vi "Msg.vi"(7 "Actor in":refnum<class "Actor.lvclass">, 11 "Actor Create Msg Strategy in":refnum<class "Actor Create Msg Strategy.lvclass">) -> (5 "Actor out":refnum<class "Actor.lvclass">)   [LabVIEW 2021, in "Actor Create.lvlib" / "Actor Create Msg Strategy.lvclass"]
uses:
  Actor Create Msg Strategy.lvclass
  jettl/Actor/Actor.lvclass
  Actor Create/Actor Create.lvclass
  b9b3c3c6-ce11-415e-ad89-e7059c446d1f.vi
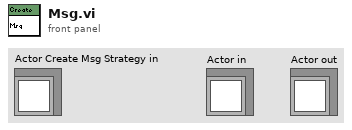
[diagram p1: front panel]
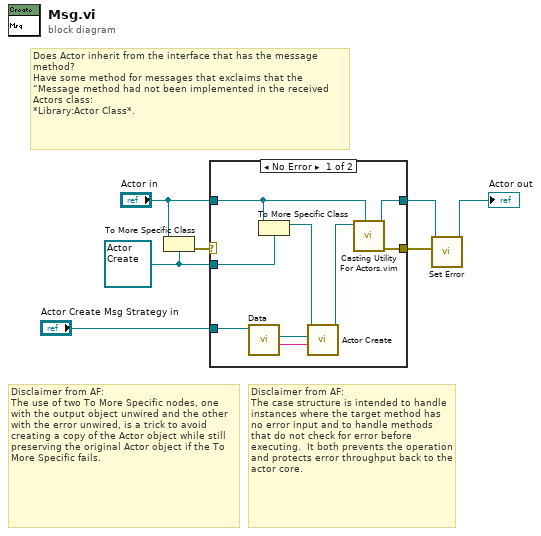
[diagram p0: block diagram]
diagram:
  w6 = refnum<class "Actor Create.lvclass"> refnum ("Create.lvlib:Create.lvclass")
  # "Disclaimer from AF:\nThe use of two To More Specific nodes, one with the output object unwired and the other with the error unwired, is a trick to avoid creating a copy of the Actor object while still preserving the original Actor object if the To More Specific fails."
  # "Disclaimer from AF:\nThe case structure is intended to handle instances where the target method has no error input and to handle methods that do not check for error before executing.  It both prevents the operation and protects error throughput back to the actor core."
  # "Does Actor inherit from the interface that has the message method?\nHave some method for messages that exclaims that the “Message method had not been implemented in the received Actors class:\n*Library:Actor Class*."
  n1 = To More Specific Class(target class=w6, reference="Actor in") -> (error out=w7:errorcluster)  [unwired: 1 in, 1 out]
  n2 = case shown="No Error" w7 {
    selector: w7 -> [_ w17]
    tunnel: [w13 w18] -> w2
    tunnel: "Actor in" -> [w12 w18]
    tunnel: w6 -> [w15 _]
    tunnel: "Actor Create Msg Strategy in" -> [w11 _]
    tunnel: [w8 w17] -> w3
    frame No Error {
      n3 = call "Data.vi"("Actor Create Msg Strategy in"=w11) -> ("Nested Alias"=w9:string, "Nested Actor"=w10:refnum<class "Actor.lvclass">)  [unwired: 9 in]
      n4 = To More Specific Class(target class=w15, reference=w12) -> (specific class reference=w16:refnum<class "Actor Create.lvclass">)  [unwired: 1 in, 1 out]
      n5 = call-dynamic "Actor Create.vi"("Nested Alias"=w9, "Nested Actor"=w10, "Actor Create in"=w16) -> ("Actor Create out"=w14:refnum<class "Actor Create.lvclass">)  [unwired: 8 in]
      n6 = call "Casting Utility For Actors.vim"("type"=w12, "Actor in"=w14) -> ("error out"=w8:errorcluster, "Actor out"=w13:refnum<class "Actor.lvclass">)  [unwired: 8 in]
    }
    frame Error {
    }
  }
  n7 = call-dynamic "Set Error.vi"("Error"=w3, "Actor in"=w2) -> ("Actor out"=→"Actor out":refnum<class "Actor.lvclass">)  [unwired: 9 in]
